vi "OE1022D_Read 1 parameter.vi"(1 "数据转换":u8[](array[numeric]), 5 "Parameter 3":u16(ring) items=["AUX1", "AUX2", "AUX3", "AUX4"], 7 "Parameter 2":u16(ring) items=["X", "Y", "R", "Theta", "Frequency", "Noise", "Xh1", "Yh1", "Rh1", "Theta h1", "Xh2", "Yh2", "Rh2", "Theta h2"], 8 "错误输入（无错误）":errorcluster, 9 "Parameter":u16(ring) items=["X", "Y", "R", "Theta", "Frequency", "Noise", "Xh1", "Yh1", "Rh1", "Theta h1", "Xh2", "Yh2", "Rh2", "Theta h2"], 10 "Channel (0: A)":u16(ring) items=["Channel A", "Channel B", "ADC"], 11 "VISA resource name":refnum<visa-resource-name>) -> (0 "error out":errorcluster, 2 "Measurement":dbl format="%.3p", 3 "VISA resource name out":refnum<visa-resource-name>)   [LabVIEW 2021]
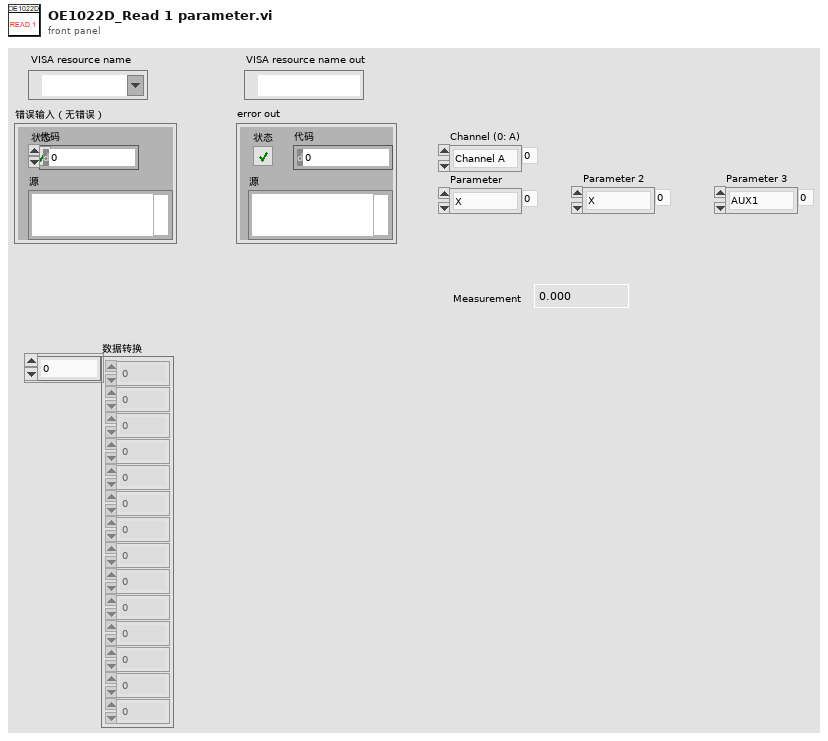
[diagram p1: front panel]
types:
  T1 = cluster{"AD1":dbl[], "AD2":dbl[], "AD3":dbl[], "AD4":dbl[]}
  T2 = cluster{"XA":dbl[], "YA":dbl[], "FrequencyA":dbl[], "NoiseA":dbl[], "Xh1A":dbl[], "Yh1A":dbl[], "Xh2A":dbl[], "Yh2A":dbl[]}
  T3 = cluster{"XB":dbl[], "YB":dbl[], "FrequencyB":dbl[], "NoiseB":dbl[], "Xh1B":dbl[], "Yh1B":dbl[], "Xh2B":dbl[], "Yh2B":dbl[], "Xh2B":dbl[]}
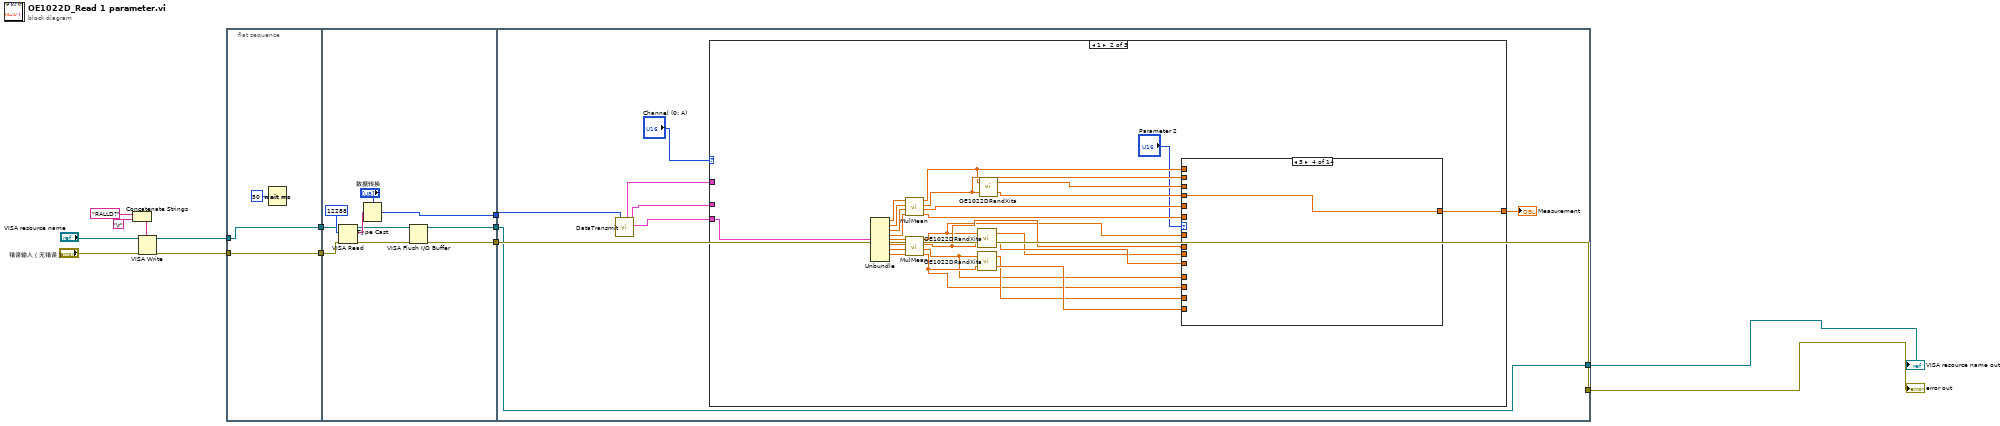
[diagram p0: block diagram]
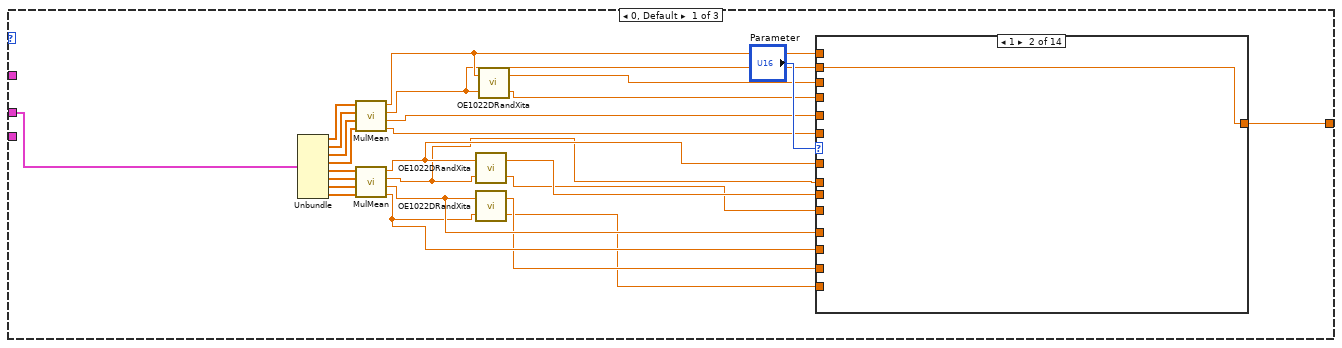
[diagram p2: hidden frame]
diagram:
  n1 = Concatenate Strings("RALLD?" ("命令输入"), "\r") -> (w13:string)
  n2 = VISA Write(VISA resource name="VISA resource name", write buffer=w13, error in (no error)="错误输入（无错误）") -> (VISA resource name out=w9:refnum<visa-resource-name>, error out=w8:errorcluster)  [unwired: 1 out]
  n3 = flat-sequence {
    tunnel: w9 -> [w15]
    tunnel: w8 -> [w16]
    tunnel: [w16] -> w7
    tunnel: [w15] -> w6
    tunnel: w7 -> [w19]
    tunnel: w6 -> [w18]
    tunnel: [w22] -> w3
    tunnel: [w21] -> w2
    tunnel: [w20] -> w1
    tunnel: w3 -> [w31]
    tunnel: w2 -> [w34]
    tunnel: w1 -> [w33]
    tunnel: [w34] -> w4
    tunnel: [w33] -> w5
    frame #0 {
      n4 = Wait (ms)(milliseconds to wait=u32 50 ("等待时间（毫秒）")) -> ()  [unwired: 1 out]
    }
    frame #1 {
      n5 = VISA Read(VISA resource name=w18, byte count=12288, error in (no error)=w19) -> (VISA resource name out=w24:refnum<visa-resource-name>, read buffer=w26:string, error out=w25:errorcluster)  [unwired: 1 out]
      n6 = Type Cast(type="数据转换", x=w26) -> (*(type *) &x=w22:u8[])
      n7 = VISA Flush I/O Buffer(VISA resource name=w24, error in (no error)=w25) -> (VISA resource name out=w20:refnum<visa-resource-name>, error out=w21:errorcluster)  [unwired: 1 in]
    }
    frame #2 {
      n8 = call <instrlib>:"DataTransmit.vi"("数据输入"=w31) -> ("输出簇ADC"=w30:T1, "输出簇A"=w29:T2, "输出簇B"=w28:T3)  [unwired: 2 in, 2 out]
      n9 = case shown="1" "Channel (0: A)" {
        tunnel: w30 -> [_ _ w120]
        tunnel: w29 -> [w51 _ _]
        tunnel: w28 -> [_ w75 _]
        tunnel: [w46 w76 w114] -> w32
        frame 0, Default {
          n10 = Unbundle(w51) -> ("XA"=w52:dbl[], "YA"=w53:dbl[], "FrequencyA"=w54:dbl[], "NoiseA"=w55:dbl[], "Xh1A"=w56:dbl[], "Yh1A"=w57:dbl[], "Xh2A"=w58:dbl[], "Yh2A"=w59:dbl[])
          n11 = call <instrlib>:"MulMean.vi"("IN 4"=w55, "IN 3"=w54, "IN 2"=w53, "IN 1"=w52) -> ("mean 4"=w40:dbl, "mean 3"=w41:dbl, "mean 2"=w49:dbl, "mean 1"=w50:dbl)  [unwired: 4 in]
          n12 = call <instrlib>:"MulMean.vi"("IN 4"=w59, "IN 3"=w58, "IN 2"=w57, "IN 1"=w56) -> ("mean 4"=w38:dbl, "mean 3"=w39:dbl, "mean 2"=w44:dbl, "mean 1"=w45:dbl)  [unwired: 4 in]
          n13 = call <instrlib>:"OE1022DRandXita.vi"("Y"=w44, "X"=w45) -> ("θ (°)"=w42:dbl, "R"=w43:dbl)
          n14 = call <instrlib>:"OE1022DRandXita.vi"("Y"=w38, "X"=w39) -> ("θ (°)"=w36:dbl, "R"=w37:dbl)
          n15 = call <instrlib>:"OE1022DRandXita.vi"("Y"=w49, "X"=w50) -> ("θ (°)"=w47:dbl, "R"=w48:dbl)
          n16 = case shown="1" "Parameter" {
            tunnel: w50 -> [w61 _ _ _ _ _ _ _ _ _ _ _ _ _]
            tunnel: w49 -> [_ w62 _ _ _ _ _ _ _ _ _ _ _ _]
            tunnel: w48 -> [_ _ w63 _ _ _ _ _ _ _ _ _ _ _]
            tunnel: w47 -> [_ _ _ w64 _ _ _ _ _ _ _ _ _ _]
            tunnel: [w61 w62 w63 w64 w65 w66 w67 w68 w69 w70 w71 w72 w73 w74] -> w46
            tunnel: w45 -> [_ _ _ _ _ _ w67 _ _ _ _ _ _ _]
            tunnel: w44 -> [_ _ _ _ _ _ _ w68 _ _ _ _ _ _]
            tunnel: w43 -> [_ _ _ _ _ _ _ _ w69 _ _ _ _ _]
            tunnel: w42 -> [_ _ _ _ _ _ _ _ _ w70 _ _ _ _]
            tunnel: w41 -> [_ _ _ _ w65 _ _ _ _ _ _ _ _ _]
            tunnel: w40 -> [_ _ _ _ _ w66 _ _ _ _ _ _ _ _]
            tunnel: w39 -> [_ _ _ _ _ _ _ _ _ _ w71 _ _ _]
            tunnel: w38 -> [_ _ _ _ _ _ _ _ _ _ _ w72 _ _]
            tunnel: w37 -> [_ _ _ _ _ _ _ _ _ _ _ _ w73 _]
            tunnel: w36 -> [_ _ _ _ _ _ _ _ _ _ _ _ _ w74]
            frame 0, Default {
            }
            frame 1 {
            }
            frame 2 {
            }
            frame 3 {
            }
            frame 4 {
            }
            frame 5 {
            }
            frame 6 {
            }
            frame 7 {
            }
            frame 8 {
            }
            frame 9 {
            }
            frame 10 {
            }
            frame 11 {
            }
            frame 12 {
            }
            frame 13 {
            }
          }
        }
        frame 1 {
          n17 = Unbundle(w75) -> ("XB"=w85:dbl[], "YB"=w84:dbl[], "FrequencyB"=w83:dbl[], "NoiseB"=w82:dbl[], "Xh1B"=w81:dbl[], "Yh1B"=w80:dbl[], "Xh2B"=w79:dbl[], "Yh2B"=w78:dbl[])  [unwired: 1 out]
          n18 = call <instrlib>:"MulMean.vi"("IN 4"=w82, "IN 3"=w83, "IN 2"=w84, "IN 1"=w85) -> ("mean 4"=w95:dbl, "mean 3"=w94:dbl, "mean 2"=w87:dbl, "mean 1"=w86:dbl)  [unwired: 4 in]
          n19 = call <instrlib>:"MulMean.vi"("IN 4"=w78, "IN 3"=w79, "IN 2"=w80, "IN 1"=w81) -> ("mean 4"=w97:dbl, "mean 3"=w96:dbl, "mean 2"=w91:dbl, "mean 1"=w90:dbl)  [unwired: 4 in]
          n20 = call <instrlib>:"OE1022DRandXita.vi"("Y"=w91, "X"=w90) -> ("θ (°)"=w93:dbl, "R"=w92:dbl)
          n21 = call <instrlib>:"OE1022DRandXita.vi"("Y"=w97, "X"=w96) -> ("θ (°)"=w99:dbl, "R"=w98:dbl)
          n22 = call <instrlib>:"OE1022DRandXita.vi"("Y"=w87, "X"=w86) -> ("θ (°)"=w89:dbl, "R"=w88:dbl)
          n23 = case shown="3" "Parameter 2" {
            tunnel: w86 -> [w100 _ _ _ _ _ _ _ _ _ _ _ _ _]
            tunnel: w87 -> [_ w101 _ _ _ _ _ _ _ _ _ _ _ _]
            tunnel: w88 -> [_ _ w102 _ _ _ _ _ _ _ _ _ _ _]
            tunnel: w89 -> [_ _ _ w103 _ _ _ _ _ _ _ _ _ _]
            tunnel: [w100 w101 w102 w103 w104 w105 w106 w107 w108 w109 w110 w111 w112 w113] -> w76
            tunnel: w90 -> [_ _ _ _ _ _ w106 _ _ _ _ _ _ _]
            tunnel: w91 -> [_ _ _ _ _ _ _ w107 _ _ _ _ _ _]
            tunnel: w92 -> [_ _ _ _ _ _ _ _ w108 _ _ _ _ _]
            tunnel: w93 -> [_ _ _ _ _ _ _ _ _ w109 _ _ _ _]
            tunnel: w94 -> [_ _ _ _ w104 _ _ _ _ _ _ _ _ _]
            tunnel: w95 -> [_ _ _ _ _ w105 _ _ _ _ _ _ _ _]
            tunnel: w96 -> [_ _ _ _ _ _ _ _ _ _ w110 _ _ _]
            tunnel: w97 -> [_ _ _ _ _ _ _ _ _ _ _ w111 _ _]
            tunnel: w98 -> [_ _ _ _ _ _ _ _ _ _ _ _ w112 _]
            tunnel: w99 -> [_ _ _ _ _ _ _ _ _ _ _ _ _ w113]
            frame 0, Default {
            }
            frame 1 {
            }
            frame 2 {
            }
            frame 3 {
            }
            frame 4 {
            }
            frame 5 {
            }
            frame 6 {
            }
            frame 7 {
            }
            frame 8 {
            }
            frame 9 {
            }
            frame 10 {
            }
            frame 11 {
            }
            frame 12 {
            }
            frame 13 {
            }
          }
        }
        frame 2 {
          n24 = Unbundle By Name(w120) -> ("AD1"=w124:dbl[], "AD2"=w123:dbl[], "AD3"=w122:dbl[], "AD4"=w121:dbl[])
          n25 = call <instrlib>:"MulMean.vi"("IN 4"=w121, "IN 3"=w122, "IN 2"=w123, "IN 1"=w124) -> ("mean 4"=w115:dbl, "mean 3"=w116:dbl, "mean 2"=w117:dbl, "mean 1"=w118:dbl)  [unwired: 4 in]
          n26 = case shown="0, Default" "Parameter 3" {
            tunnel: w118 -> [w125 _ _ _]
            tunnel: w117 -> [_ w126 _ _]
            tunnel: w116 -> [_ _ w127 _]
            tunnel: w115 -> [_ _ _ w128]
            tunnel: [w125 w126 w127 w128] -> w114
            frame 0, Default {
            }
            frame 1 {
            }
            frame 2 {
            }
            frame 3 {
            }
          }
        }
      }
      "Measurement" <- w32
    }
  }
  "VISA resource name out" <- w5
  "error out" <- w4
